vi "CalculateUnbalanceFactor.vi"(6 "Calculation Cache In":T1, 8 "error in (no error)":errorcluster, 11 "voltage waveforms":waveform(dbl)[](array[waveform])) -> (0 "error out":errorcluster, 3 "derating factor":sgl, 4 "Calculation Cache Out":T1)   [LabVIEW 2017, in "McsaAnalysisFunctions.lvlib"]
uses:
  <vilib>/addons/InsightCM/Utilities/Analysis/MCSA/McsaAnalysisFunctions.lvlib
  <vilib>/addons/InsightCM/Utilities/Analysis/MCSA/controls/MotorCalculationCache.ctl
  <vilib>/addons/Electrical Power/Basic/Measurement/subVIs/basic_Power Value.ctl
  <vilib>/addons/InsightCM/Utilities/Analysis/MCSA/controls/TorqueLoadEfficiency.ctl
  <vilib>/addons/Electrical Power/Basic/NI_EP_Basic.lvlib
  <vilib>/addons/Electrical Power/Motor Monitoring/NI_EP_Motor Monitoring.lvlib
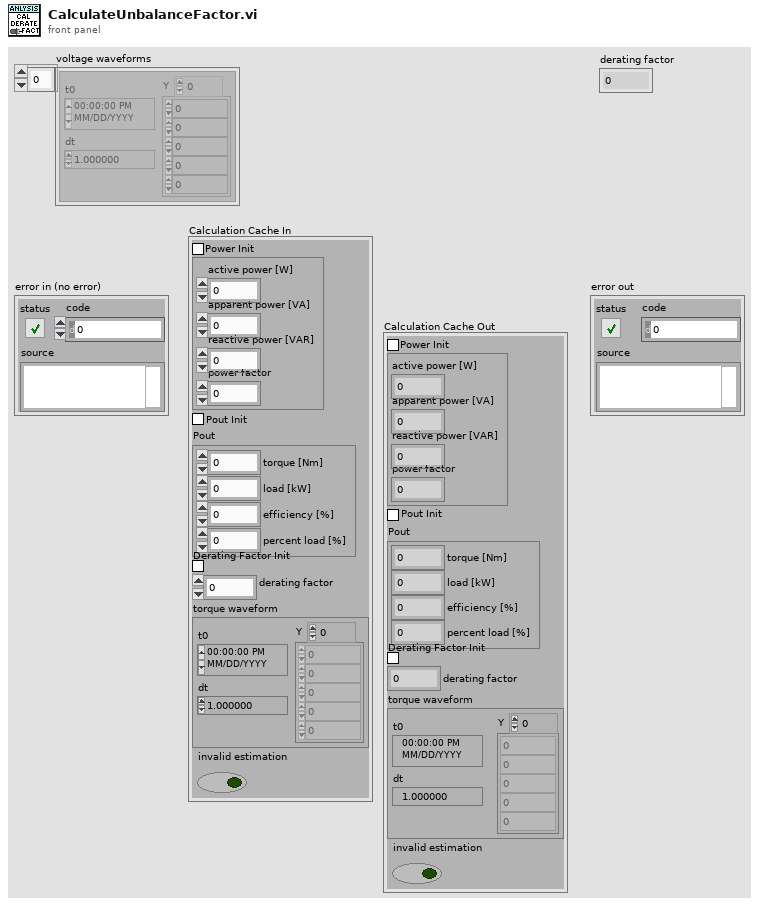
[diagram p1: front panel]
types:
  T1 = typedef "McsaAnalysisFunctions.lvlib/MotorCalculationCache.ctl" = cluster{"Power Init":bool, "power value":T2, "Pout Init":bool, "Pout":T3, "Derating Factor Init":bool, "derating factor":sgl, "torque waveform":waveform(dbl), "invalid estimation":bool}
  T2 = typedef "NI_EP_Basic.lvlib/basic_Power Value.ctl" = cluster{"active power [W]":dbl, "apparent power [VA]":dbl, "reactive power [VAR]":dbl, "power factor":dbl}
  T3 = typedef "McsaAnalysisFunctions.lvlib/TorqueLoadEfficiency.ctl" = cluster{"torque [Nm]":dbl, "load [kW]":dbl, "efficiency [%]":dbl, "percent load [%]":dbl}
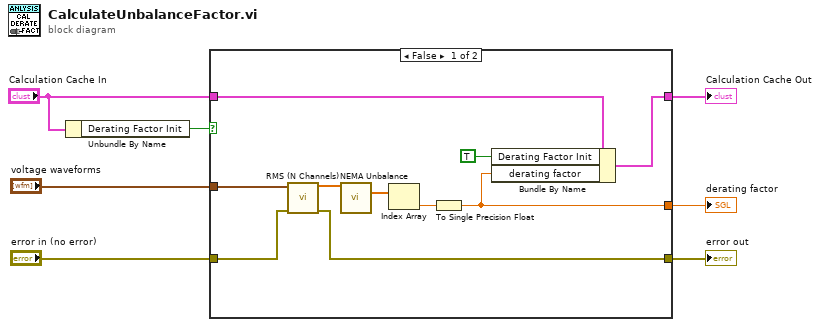
[diagram p0: block diagram]
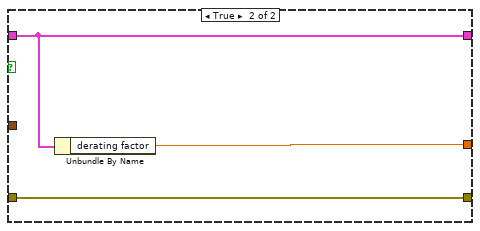
[diagram p2: hidden frame]
diagram:
  n1 = Unbundle By Name("Calculation Cache In") -> ("Derating Factor Init"=w2:bool)
  n2 = case shown="False" w2 {
    tunnel: "voltage waveforms" -> [w8 _]
    tunnel: [w17 w19] -> w6
    tunnel: "error in (no error)" -> [w16 w19]
    tunnel: [w15 w20] -> w4
    tunnel: "Calculation Cache In" -> [w14 w20]
    tunnel: [w13 w18] -> w1
    frame False {
      n3 = call <vilib>:"RMS (N Channels).vi"("error in (no error)"=w16, "waveforms"=w8) -> ("error out"=w17:errorcluster, "RMS values"=w12:dbl[])  [unwired: 8 in]
      n4 = call <vilib>:"NEMA Unbalance.vi"("voltage RMS values"=w12) -> ("unbalance derating factors"=w11:dbl[])  [unwired: 12 in, 2 out]
      n5 = Index Array(array=w11) -> (element=w9:dbl)  [unwired: 1 in]
      n6 = To Single Precision Float(number=w9) -> (single precision float=w13:sgl)
      n7 = Bundle By Name(cluster=w14, "Derating Factor Init"=TRUE ("Unbalance Init"), "derating factor"=w13) -> (w15:T1)
    }
    frame True {
      n8 = Unbundle By Name(w20) -> ("derating factor"=w18:sgl)
    }
  }
  "error out" <- w6
  "Calculation Cache Out" <- w4
  "derating factor" <- w1
